vi "Create Serial Slave.vi"(4 "flow control":u16(ring) items=["None", "XON/XOFF", "RTS/CTS", "XON/XOFF & RTS/CTS", "DTR/DSR", "XON/XOFF & DTR/DSR"], 5 "serial type":enum16{"RTU", "ASCII"}(ring), 6 "parity (even)":u16(ring)=2 items=["None", "Odd", "Even", "Mark", "Space"], 7 "unit ID":u8=1, 8 "error in":errorcluster, 9 "device data model":refnum<class "Device Data Model.lvclass">, 10 "baud rate (9600)":u32=9600, 11 "VISA resource name":refnum<visa-resource-name>) -> (0 "error out":errorcluster, 3 "serial slave instance":refnum<class "Modbus Slave.lvclass">)   [LabVIEW 2014, in "MyLib.lvlib" / "API Main.lvlib"]
doc: "Creates a standard TCP slave with an IP ADU. If the data model input is unwired, a standard data model will be initialized and used. If the input is wired, the code will check to make sure that it is not the default value for the class (it should be initialized). If the default value of the class is wired, the standard model will be initialized and used."
uses:
  API Main.lvlib
  Slave/Modbus Slave.lvclass
  Data Model/Device Data Model.lvclass
  Transmission Data Unit/RTU/RTU Data Unit.lvclass
  Transmission Data Unit/RTU/RTU Data Unit.lvclass/RTU Data Unit.ctl
  Transmission Data Unit/ASCII/ASCII Data Unit.lvclass
  Transmission Data Unit/Transmission Data Unit.lvclass/Transmission Data Unit.ctl
  Network Protocol/Network Slave/Serial/Serial Slave.lvclass
  Standard Data Model/Standard Data Model.lvclass
  Data Model/Device Data Model.lvclass/Device Data Model.ctl
  Network Protocol/Network Slave/Serial/Serial Slave.lvclass/Serial Slave.ctl
  Slave/Modbus Slave.lvclass/Modbus Slave.ctl
  Modbus API.lvclass/Modbus API.ctl
  Network Protocol/Network Slave/Serial/Write Baud Rate.vi
  Network Protocol/Network Slave/Serial/Write Flow Control.vi
  Network Protocol/Network Slave/Serial/Write Parity.vi
  Network Protocol/Network Slave/Serial/Write VISA resource name.vi
  Network Protocol/Network Slave/Serial/Write Serial Data Unit.vi
  Data Model/Read Initialized.vi
  <vilib>/Utility/error.llb/Clear Errors.vi
  Modbus API.lvclass
  Transmission Data Unit/Transmission Data Unit.lvclass
panel:
  # "disable parity disallowed by mbspec"
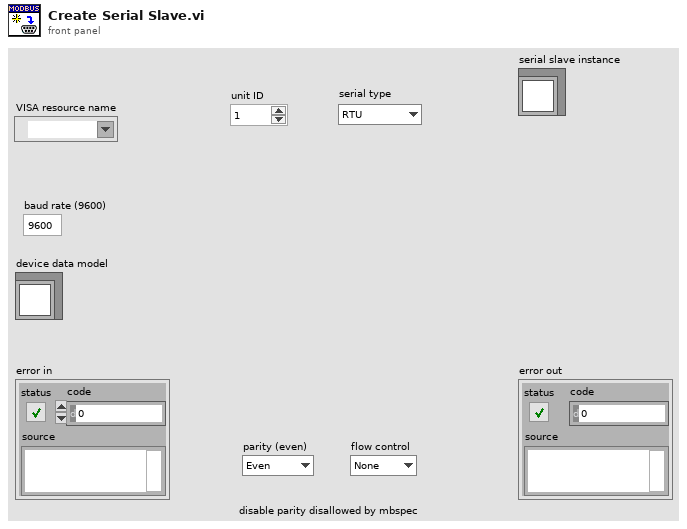
[diagram p1: front panel]
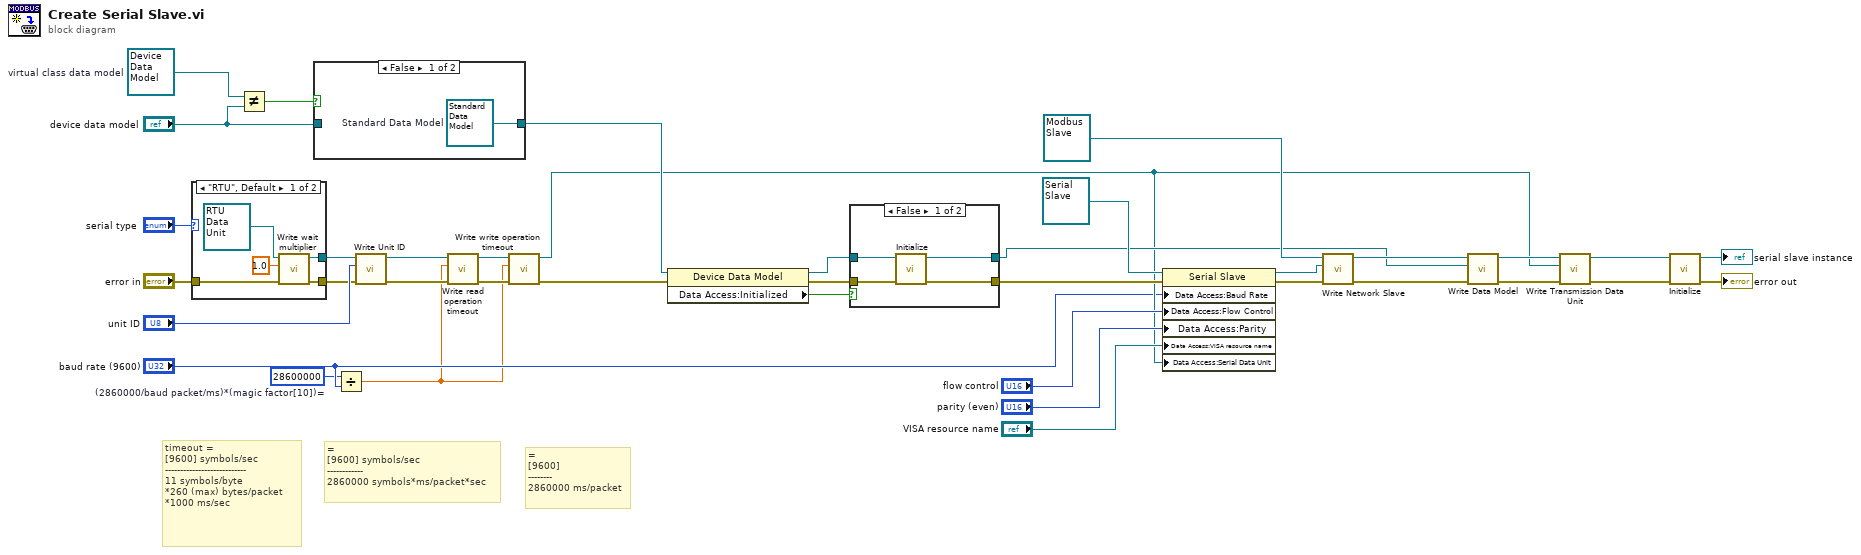
[diagram p0: block diagram]
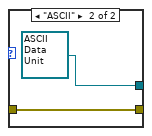
[diagram p4: hidden frame]
diagram:
  w5 = u32 28600000  # (2860000/baud packet/ms)*(magic factor[10])=
  w29 = refnum<class "Device Data Model.lvclass"> refnum  # virtual class data model
  # "=\n[9600]\n--------\n2860000 ms/packet"
  # "=\n[9600] symbols/sec\n------------\n2860000 symbols*ms/packet*sec"
  # "timeout =\n[9600] symbols/sec\n---------------------------\n11 symbols/byte\n*260 (max) bytes/packet\n*1000 ms/sec"
  n1 = case shown="\"RTU\", Default" "serial type" {
    tunnel: [w43 w45] -> w3
    tunnel: "error in" -> [w42 w45]
    tunnel: [w39 refnum<class "ASCII Data Unit.lvclass"> refnum ("ASCII Data Unit")] -> w1
    frame "RTU", Default {
      n2 = call "Write wait multiplier.vi"("error in (no error)"=w42, "wait multiplier"=sgl 1.0, "RTU Data Unit in"=refnum<class "RTU Data Unit.lvclass"> refnum ("RTU Data Unit")) -> ("error out"=w43:errorcluster, "RTU Data Unit out"=w39:refnum<class "RTU Data Unit.lvclass">)  [unwired: 7 in]
    }
    frame "ASCII" {
    }
  }
  n3 = Not Equal?(x=w29, y="device data model") -> (x != y?=w28:bool)
  n4 = case shown="False" w28 {
    tunnel: "device data model" -> [_ w47]
    tunnel: [w46 w47] -> w25
    frame False {
      w46 = refnum<class "Standard Data Model.lvclass"> refnum  # Standard Data Model
    }
    frame True {
    }
  }
  n5 = Divide(x=w5, y="baud rate (9600)") -> (x/y=w4:dbl)
  n6 = call "Write Unit ID.vi"("error in"=w3, "unit ID"="unit ID", "transmission data unit in"=w1) -> ("error out"=w7:errorcluster, "transmission data unit out"=w12:refnum<class "Serial Data Unit.lvclass">)  [unwired: 7 in]
  n7 = call "Write read operation timeout.vi"("error in (no error)"=w7, "read operation timeout"=w4, "transmission data unit in"=w12) -> ("error out"=w8:errorcluster, "transmission data unit out"=w11:refnum<class "Serial Data Unit.lvclass">)  [unwired: 7 in]
  n8 = call "Write write operation timeout.vi"("error in (no error)"=w8, "write operation timeout"=w4, "transmission data unit in"=w11) -> ("error out"=w9:errorcluster, "transmission data unit out"=w10:refnum<class "Serial Data Unit.lvclass">)  [unwired: 7 in]
  n9 = property class="Device Data Model"(reference=w25, error in=w9) -> (reference out=w31:refnum<class "Device Data Model.lvclass">, error out=w32:errorcluster, "Data Access:Initialized"=w30:bool)
  n10 = case shown="False" w30 {
    tunnel: w32 -> [w51 w53]
    tunnel: [w50 w53] -> w26
    tunnel: [w49 w52] -> w15
    tunnel: w31 -> [w48 w52]
    frame False {
      n11 = call-dynamic "Initialize.vi"("error in"=w51, "device data model in"=w48) -> ("error out"=w50:errorcluster, "device data model out"=w49:refnum<class "Device Data Model.lvclass">)  [unwired: 8 in]
    }
    frame True {
    }
  }
  n12 = property class="Serial Slave"(reference=refnum<class "Serial Slave.lvclass"> refnum ("Serial Slave"), error in=w26, "Data Access:Baud Rate"="baud rate (9600)", "Data Access:Flow Control"="flow control", "Data Access:Parity"="parity (even)", "Data Access:VISA resource name"="VISA resource name", "Data Access:Serial Data Unit"=w10) -> (reference out=w20:refnum<class "Serial Slave.lvclass">, error out=w19:errorcluster)
  n13 = call "Write Network Slave.vi"("error in"=w19, "network slave"=w20, "Modbus slave in"=refnum<class "Modbus Slave.lvclass"> refnum ("Modbus Slave")) -> ("error out"=w18:errorcluster, "Modbus slave out"=w17:refnum<class "Modbus Slave.lvclass">)  [unwired: 7 in]
  n14 = call "Write Data Model.vi"("error in"=w18, "Device Data Model"=w15, "Modbus slave in"=w17) -> ("error out"=w21:errorcluster, "Modbus slave out"=w22:refnum<class "Modbus Slave.lvclass">)  [unwired: 7 in]
  n15 = call "Write Transmission Data Unit.vi"("error in"=w21, "transmission data unit"=w10, "Modbus instance in"=w22) -> ("error out"=w23:errorcluster, "Modbus instance out"=w24:refnum<class "Modbus Slave.lvclass">)  [unwired: 7 in]
  n16 = call-dynamic "Initialize.vi"("error in"=w23, "Modbus slave in"=w24) -> ("error out"=→"error out":errorcluster, "Modbus slave out"=→"serial slave instance":refnum<class "Modbus Slave.lvclass">)  [unwired: 8 in]
